vi "CIE-Config.vi"(0 "Cal Stimulus":T2, 5 "Speaker":T3, 7 "Weighted":T1 {"WF" items=["Chirp", "Noise"]}, 9 "Fish shaker":bool, 11 "error in (no error)":errorcluster) -> (3 "Stimulus waveform":cluster{i32, dbl, dbl[]}, 4 "Stimulus":dbl[](array[numeric]), 6 "Cal Spec Out":T2={"Min Freq (Hz)"=50.0, "Max Freq (Hz)"=50000.0, "Freq Step (Hz)"=50.0, "Waveform"=enum."Chirp", "Attenuation (dB)"=20.0, "Sample Rate (Hz)"=100000.0}, 8 "Mic Avg":dbl[][](array[numeric]), 10 "dt (ms)":dbl, 13 "df (Hz)":dbl, 15 "error out":errorcluster)   [LabVIEW 2020]
uses:
  Type Defs/Cal Stimulus.ctl
  Utility VIs/Type Defs/Speaker ring.ctl
  Type Defs/ACal-Multiband Parameters.ctl
  Misc VIs/Connection Manager/Type Defs/Input sources.ctl
  Misc VIs/Connection Manager/Type Defs/Output sources.ctl
  PXI DAQ VIs/DAQ Engine VIs/AO Gain and Multiplier VIs/PXI Multipliers to AO Gains (1D).vi
  PXI DAQ VIs/TDT VIs/TDT-Signal Bank Action.ctl
  Utility VIs/Math VIs/dB to Linear (scalar).vi
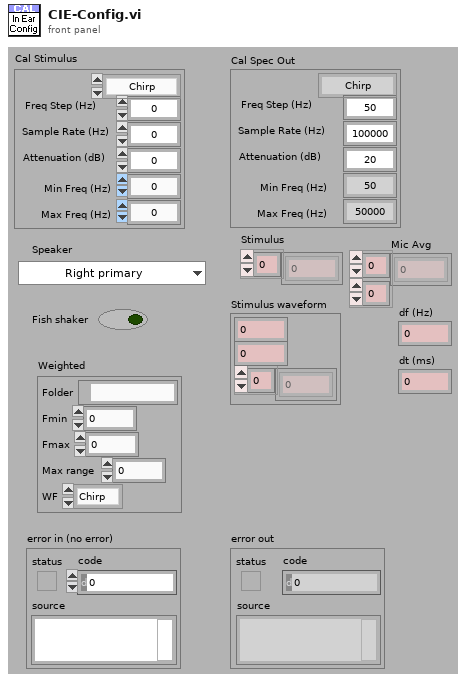
[diagram p1: front panel]
types:
  T1 = typedef "ACal-Multiband Parameters.ctl" = cluster{"Folder":path, "Fmin":dbl, "Fmax":dbl, "Max range":dbl, "WF":u16}
  T2 = typedef "Cal Stimulus.ctl" = cluster{"Min Freq (Hz)":dbl, "Max Freq (Hz)":dbl, "Freq Step (Hz)":dbl, "Waveform":enum16{"Chirp", "Weighted"}, "Attenuation (dB)":dbl, "Sample Rate (Hz)":dbl}
  T3 = typedef "Speaker ring.ctl" = enum16{"Right primary", "Right secondary", "Left primary", "Left secondary"}
  T4 = typedef "TDT-Signal Bank Action.ctl" = enum16{"Init", "Write", "Read", "Rewrite", "Reset", "Recycle", "Ramp up", "Ramp down", "Zero"}
  T5 = typedef "Output sources.ctl" = u16
  T6 = typedef "Input sources.ctl" = u16
  T7 = typedef "TDT-Device Config.ctl" = cluster{"Output":T8, "Input":T10}
  T8 = typedef "TDT-Output source.ctl" = cluster{"Device":T9, "Num":i32}
  T9 = typedef "TDT-Device ID.ctl" = enum16{"None", "PA5", "RP2", "RL2", "RA16", "RV8", "RX5", "RX6", "RX7", "RX8", "RZ2", "RZ5", "RZ6"}
  T10 = typedef "TDT-Input source.ctl" = enum16{"Front Panel", "RA4LI", "RA16LI"}
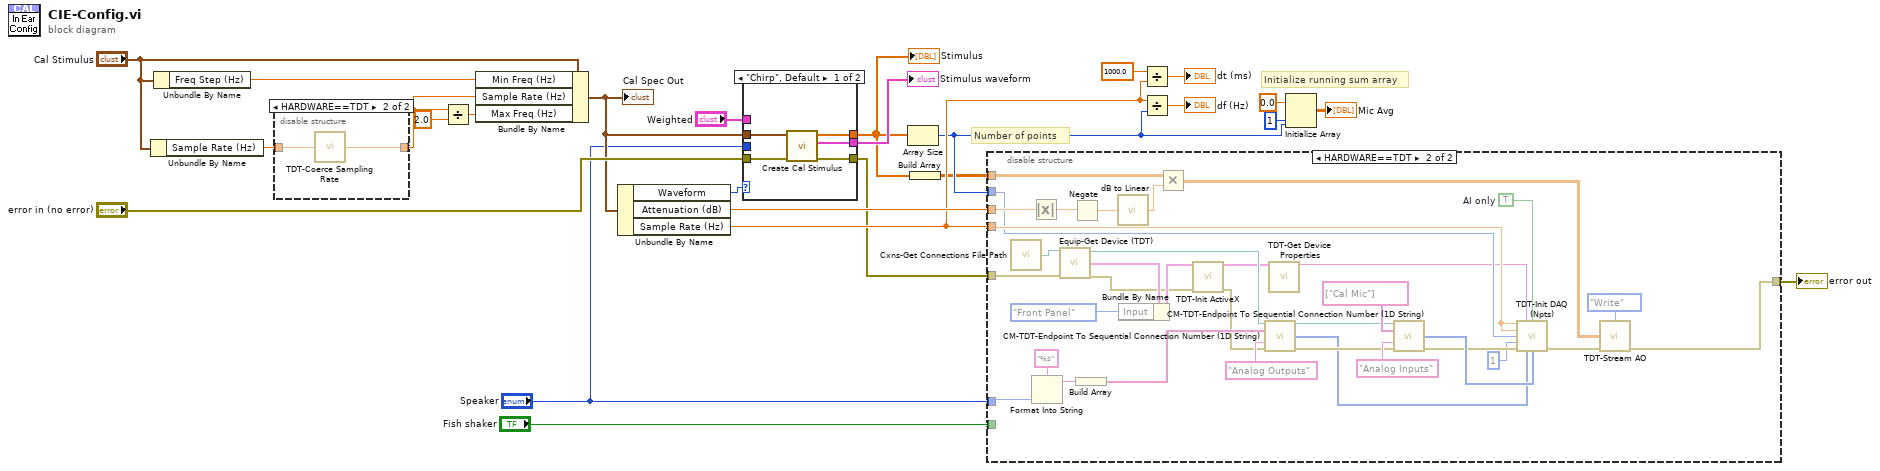
[diagram p0: block diagram]
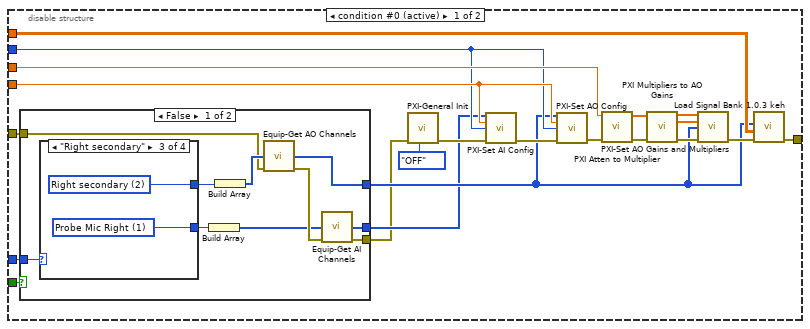
[diagram p3: hidden frame]
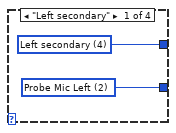
[diagram p4: hidden frame]
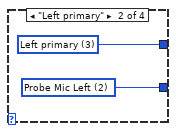
[diagram p5: hidden frame]
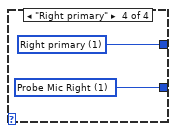
[diagram p6: hidden frame]
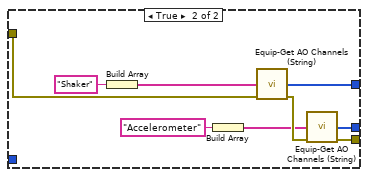
[diagram p7: hidden frame]
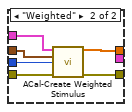
[diagram p8: hidden frame]
diagram:
  # "Number of points"
  # "Initialize running sum array"
  n1 = Unbundle By Name("Cal Stimulus") -> ("Sample Rate (Hz)"=w1:dbl)
  n2 = Unbundle By Name("Cal Stimulus") -> ("Freq Step (Hz)"=w12:dbl)
  n3 = disable-structure shown="HARDWARE==TDT" {
    disable-tunnel: [w27 w29] -> w3
    disable-tunnel: w1 -> [w27 w28]
    frame condition #0 (active) {
    }
    frame condition #1 {
      n4 = call "TDT-Coerce Sampling Rate.vi"("Fs (Hz)"=w28) -> ("Coerced"=w29:dbl)
    }
  }
  n5 = Divide(x=w3, y=2.0) -> (x/y=w11:dbl)
  n6 = Bundle By Name(cluster="Cal Stimulus", "Min Freq (Hz)"=w12, "Sample Rate (Hz)"=w3, "Max Freq (Hz)"=w11) -> (w7:T2)
  "Cal Spec Out" <- w7
  n7 = Unbundle By Name(w7) -> ("Waveform"=w6:enum16{"Chirp", "Weighted"}, "Attenuation (dB)"=w24:dbl, "Sample Rate (Hz)"=w15:dbl)
  n8 = case shown="\"Chirp\", Default" w6 {
    tunnel: [w34 _] -> w26
    tunnel: [w33 w38] -> w25
    tunnel: "error in (no error)" -> [w32 w39]
    tunnel: [w31 w37] -> w8
    tunnel: w7 -> [w30 w35]
    tunnel: "Weighted" -> [_ w40]
    tunnel: "Speaker" -> [_ w36]
    frame "Chirp", Default {
      n9 = call "Create Cal Stimulus.vi"("error in (no error)"=w32, "Cal Stimulus"=w30) -> ("error out"=w31:errorcluster, "Stimulus waveform"=w34:cluster{i32, dbl, dbl[]}, "Stimulus"=w33:dbl[])  [unwired: 7 in]
    }
    frame "Weighted" {
      n10 = call "ACal-Create Weighted Stimulus.vi"("Weighted"=w40, "Cal Stimulus"=w35, "Speaker"=w36, "error in (no error)"=w39) -> ("Stimulus"=w38:dbl[], "error out"=w37:errorcluster)  [unwired: 10 in]
    }
  }
  "Stimulus" <- w25
  "Stimulus waveform" <- w26
  n11 = Array Size(array=w25) -> (size(s)=w14:i32)
  n12 = Build Array(w25) -> (w13:dbl[][])
  n13 = disable-structure shown="HARDWARE==TDT" {
    disable-tunnel: w24 -> [w59 w116]
    disable-tunnel: [w58 w113] -> w16
    disable-tunnel: w15 -> [w51 w105]
    disable-tunnel: w14 -> [w50 w103]
    disable-tunnel: w13 -> [w48 w112]
    disable-tunnel: "Fish shaker" -> [w46 _]
    disable-tunnel: w8 -> [w43 w101]
    disable-tunnel: "Speaker" -> [w41 w96]
    frame condition #0 (active) {
      n14 = case shown="False" w46 {
        tunnel: [w64 w84] -> w45
        tunnel: [w65 w88] -> w44
        tunnel: w41 -> [w71 _]
        tunnel: w43 -> [w63 w85]
        tunnel: [w62 w87] -> w42
        frame False {
          n15 = case shown="\"Right secondary\"" w71 {
            tunnel: [w73 w75 w77 w79] -> w67
            tunnel: [w72 w74 w76 w78] -> w66
            frame "Left secondary" {
              w73 = T5 4 items=["--unused--", "Right primary", "Right secondary", "Left primary", "Left secondary", "Shocks", "Startle", "Background"] ("Ring")
              w72 = T6 2 items=["--unused--", "Probe Mic Right", "Probe Mic Left", "Cal Mic", "ABR", "CAP Right", "CAP Left", "Startle piezo", "Temperature", "Heart rate"] ("Ring")
            }
            frame "Left primary" {
              w75 = T5 3 items=["--unused--", "Right primary", "Right secondary", "Left primary", "Left secondary", "Shocks", "Startle", "Background"] ("Ring")
              w74 = T6 2 items=["--unused--", "Probe Mic Right", "Probe Mic Left", "Cal Mic", "ABR", "CAP Right", "CAP Left", "Startle piezo", "Temperature", "Heart rate"] ("Ring")
            }
            frame "Right secondary" {
              w77 = T5 2 items=["--unused--", "Right primary", "Right secondary", "Left primary", "Left secondary", "Shocks", "Startle", "Background"] ("Ring")
              w76 = T6 1 items=["--unused--", "Probe Mic Right", "Probe Mic Left", "Cal Mic", "ABR", "CAP Right", "CAP Left", "Startle piezo", "Temperature", "Heart rate"] ("Ring")
            }
            frame "Right primary" {
              w79 = T5 1 items=["--unused--", "Right primary", "Right secondary", "Left primary", "Left secondary", "Shocks", "Startle", "Background"] ("Ring")
              w78 = T6 1 items=["--unused--", "Probe Mic Right", "Probe Mic Left", "Cal Mic", "ABR", "CAP Right", "CAP Left", "Startle piezo", "Temperature", "Heart rate"] ("Ring")
            }
          }
          n16 = Build Array(w66) -> (w69:T6[])
          n17 = Build Array(w67) -> (w68:T5[])
          n18 = call "Equip-Get AO Channels.vi"("Outputs"=w68, "error in (no error)"=w63) -> ("AO Channels"=w64:i32[], "error out"=w70:errorcluster)  [unwired: 12 in]
          n19 = call "Equip-Get AI Channels.vi"("Inputs"=w69, "error in (no error)"=w70) -> ("AI Channels"=w65:i32[], "error out"=w62:errorcluster)  [unwired: 12 in]
        }
        frame True {
          n20 = Build Array("Shaker") -> (w82:string[])
          n21 = Build Array("Accelerometer") -> (w80:string[])
          n22 = call "Equip-Get AO Channels (String).vi"("Channel Names"=w82, "error in (no error)"=w85) -> ("AO Channels"=w84:i32[], "error out"=w86:errorcluster)  [unwired: 12 in]
          n23 = call "Equip-Get AO Channels (String).vi"("Channel Names"=w80, "error in (no error)"=w86) -> ("AO Channels"=w88:i32[], "error out"=w87:errorcluster)  [unwired: 12 in]
        }
      }
      n24 = call "PXI-General Init.vi"("Double Buffer Mode"=enum32{"OFF", "ENABLED", "FORCED"}."OFF", "error in (no error)"=w42) -> ("error out"=w54:errorcluster)  [unwired: 9 in]
      n25 = call "PXI-Set AI Config.vi"("AI Channels"=w44, "Sampling Rate (Hz)"=w51, "Buffer Size"=w50, "error in (no error)"=w54) -> ("error out"=w52:errorcluster)  [unwired: 11 in]
      n26 = call "PXI-Set AO Config.vi"("AO Channels"=w45, "Sampling Rate (Hz)"=w51, "Buffer Size"=w50, "error in (no error)"=w52) -> ("error out"=w53:errorcluster)  [unwired: 11 in]
      n27 = call "PXI Atten to Multiplier.vi"("error in (no error)"=w53, "Attenuation"=w59) -> ("error out"=w61:errorcluster, "Multiplier setting"=w60:dbl[])  [unwired: 8 in]
      n28 = call-poly "PXI Multipliers to AO Gains.vi"("Multipliers in"=w60, "error in (no error)"=w61) -> ("Multipliers out"=w56:dbl[], "Gains"=w55:dbl[], "error out"=w57:errorcluster)  [unwired: 11 in]
      n29 = call "PXI-Set AO Gains and Multipliers.vi"("Multipliers"=w56, "Gains"=w55, "AO Channels"=w45, "error in (no error)"=w57) -> ("error out"=w49:errorcluster)  [unwired: 11 in]
      n30 = call "Load Signal Bank 1.0.3 keh.vi"("error in (no error)"=w49, "Input array"=w48, "Active AO Array"=w45) -> ("error out"=w58:errorcluster)  [unwired: 6 in, 2 out]
    }
    frame condition #1 {
      w107 = TRUE  # AI only
      n31 = call "Cxns-Get Connections File Path.vi"() -> ("Path Out"=w102:path)  [unwired: 1 in]
      n32 = Absolute Value(x=w116) -> (abs(x)=w115:dbl)
      n33 = Format Into String(format string="%s", w96) -> (resulting string=w94:string)  [unwired: 2 in, 1 out]
      n34 = call "Equip-Get Device (TDT).vi"("Path In"=w102, "error in (no error)"=w101) -> ("Path Out"=w98:path, "TDT-Device Config"=w99:T7, "error out"=w90:errorcluster)  [unwired: 11 in]
      n35 = Negate(x=w115) -> (-x=w117:dbl)
      n36 = Build Array(w94) -> (w93:string[])
      n37 = call-poly "dB to Linear.vi"("dB"=w117) -> ("linear"=w111:dbl)
      n38 = Bundle By Name(cluster=w99, "Input"=enum16{"Front Panel", "RA4LI", "RA16LI"}."Front Panel") -> (w92:T7)
      n39 = Multiply(x=w112, y=w111) -> (x*y=w110:dbl[][])
      n40 = call "TDT-Init ActiveX.vi"("TDT-Device Config"=w92, "error in (no error)"=w90) -> ("TDT-Device Config out"=w91:T7, "error out"=w89:errorcluster)  [unwired: 10 in, 2 out]
      n41 = call "CM-TDT-Endpoint To Sequential Connection Number (1D String).vi"("Path In"=w98, "Endpoints"=w93, "Section"="Analog Outputs", "error in (no error)"=w89) -> ("Path Out"=w121:path, "SeqCxnNum"=w106:i32[], "error out"=w120:errorcluster)  [unwired: 9 in]
      n42 = call "TDT-Get Device Properties.vi"("TDT-Device Config"=w91) -> ("Circuit File"=w97:string)  [unwired: 9 in, 5 out]
      n43 = call "CM-TDT-Endpoint To Sequential Connection Number (1D String).vi"("Path In"=w121, "Endpoints"=string[] ["Cal Mic"], "Section"="Analog Inputs", "error in (no error)"=w120) -> ("SeqCxnNum"=w109:i32[], "error out"=w108:errorcluster)  [unwired: 9 in, 1 out]
      n44 = call "TDT-Init DAQ (Npts).vi"("AO Fs (Hz)"=w105, "Circuit"=w97, "AI only"=w107, "AI Fs (Hz)"=w105, "Num AO Pts"=w103, "Num AO Buffers"=1, "error in (no error)"=w108, "AO Channels"=w106, "AI Channels"=w109) -> ("error out"=w114:errorcluster)  [unwired: 2 in, 4 out]
      n45 = call "TDT-Stream AO.vi"("Action"=TDT-Signal_Bank_Action."Write", "Output array"=w110, "error in (no error)"=w114) -> ("error out"=w113:errorcluster)  [unwired: 12 in]
    }
  }
  "error out" <- w16
  n46 = Divide(x=1000.0, y=w15) -> (x/y=→"dt (ms)":dbl)
  n47 = Divide(x=w15, y=w14) -> (x/y=→"df (Hz)":dbl)
  n48 = Initialize Array(0.0 ("element"), 1 ("dimension size"), w14) -> (→"Mic Avg":dbl[][])
